vi "Generate Report.vi"(8 "error in (no error)":errorcluster, 11 "Text based Communications Test in":refnum<class "Text based Communications Test.lvclass">) -> (0 "error out":errorcluster, 3 "Text based Communications Test out":refnum<class "Text based Communications Test.lvclass">)   [LabVIEW 2017, in "Text based Communications Test.lvlib" / "Text based Communications Test.lvclass"]
uses:
  Text based Communications Test.lvclass
  Text based Communications Test.lvclass/Text based Communications Test.ctl
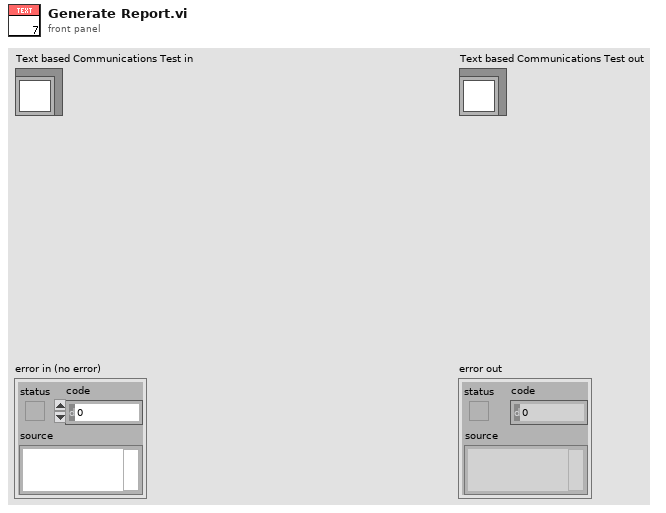
[diagram p1: front panel]
types:
  T1 = typedef "Paths.ctl" = cluster{"Data Directory":path, "Test Config Dir":path, "Error Logs":path, "Event Logs":path, "Settings.Json":path, "Reports Directory":path}
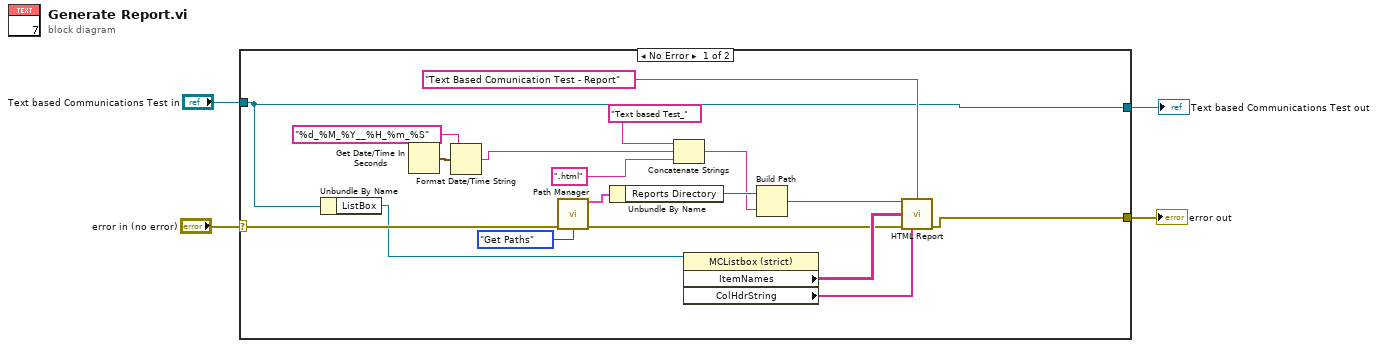
[diagram p0: block diagram]
diagram:
  n1 = case shown="No Error" "error in (no error)" {
    selector: "error in (no error)" -> [w12 w24]
    tunnel: "Text based Communications Test in" -> [w11 w23]
    tunnel: [w11 w23] -> w2
    tunnel: [w9 w24] -> w1
    frame No Error {
      n2 = Unbundle By Name(w11) -> ("ListBox"=w10:refnum<vi>)
      n3 = Get Date/Time In Seconds() -> (seconds since 1Jan1904=w7:timestamp)
      n4 = Format Date/Time String(time format string (%c)="%d_%M_%Y__%H_%m_%S", seconds (now)=w7) -> (date/time string=w5:string)  [unwired: 1 in]
      n5 = call "Path Manager.vi"("Error in (no error)"=w12, "Options"=enum16{"Get Paths", "Init Paths"}."Get Paths") -> ("Cluster"=w22:T1, "Error out"=w13:errorcluster)  [unwired: 12 in]
      n6 = Unbundle By Name(w22) -> ("Reports Directory"=w20:path)
      n7 = Concatenate Strings("Text based Test_", w5, ".html" ("string")) -> (w19:string)
      n8 = property class="MCListbox (strict)"(reference=w10) -> ("ItemNames"=w16:string[][], "ColHdrString"=w15:string[])  [unwired: 1 in, 2 out]
      n9 = Build Path(base path=w20, name or relative path=w19) -> (appended path=w18:path)
      n10 = call "HTML Report.vi"("report file path"=w18, "Column Headers"=w15, "Header"="Text Based Comunication Test - Report", "Table Data"=w16, "error in (no error)"=w13) -> ("error out"=w9:errorcluster)  [unwired: 10 in]
    }
    frame Error {
    }
  }
  "error out" <- w1
  "Text based Communications Test out" <- w2
